vi "Three_Tote_was_working_ok.vi"(11 "3_Tote_Enable":bool=TRUE) -> ()   [LabVIEW 2014]
uses:
  General_VI/Global Var.vi
panel:
  in  "Time _To_Drive_1_Tote":i32=8000
  in  "Extend_Flipper_Time":i32=500
  in  "Open_Infeed_time":i32=800
  # "Static Tunning Values"
  # "extend flipper arm was 500"
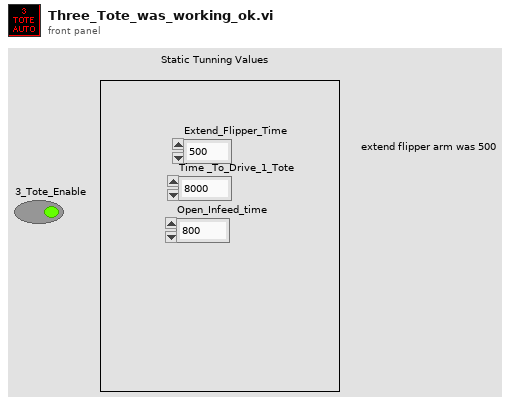
[diagram p1: front panel]
types:
  T1 = cluster{"Open_Infeed_time":i32, "Extend_Flipper_Time":i32, "Time _To_Drive_1_Tote":i32}
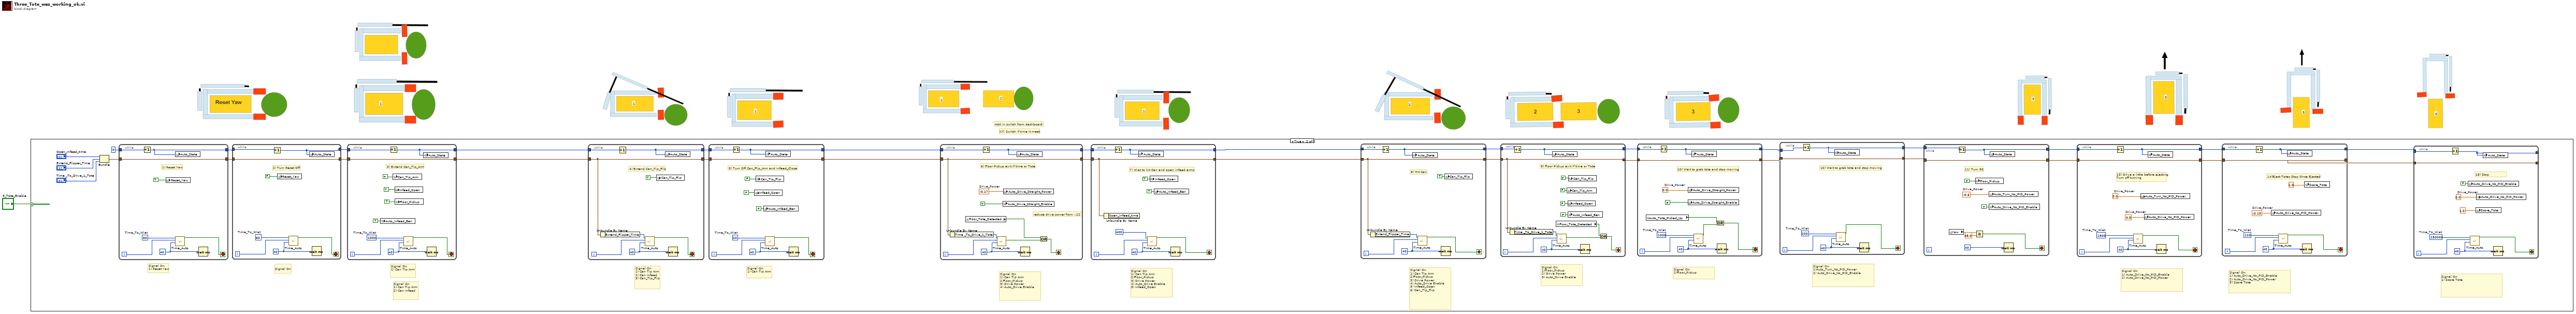
[diagram p0: block diagram]
diagram:
  # "3"
  # "3"
  # "3"
  # "3"
  # "2"
  # "2"
  # "2"
  # "1"
  # "1"
  # "1"
  # "1"
  # "Add in switch from dashboard"
  # "Kill Switch if time it meet"
  n1 = case shown="True" "3_Tote_Enable" {
    frame False {
    }
    frame True {
      # "Signal On\n1) Score Tote"
      # "Signal On\n1) Auto_Drive_No_PID_Enable\n2) Auto_Drive_No_PID_Power\n3) Score Tote"
      # "Signal On\n1) Auto_Drive_No_PID_Enable\n2) Auto_Drive_No_PID_Power"
      # "Signal On\n1)Auto_Turn_No_PID_Power\n2) Auto_Drive_No_PID_Enable"
      # "Signal On\n1)Floor_Pickup"
      # "Signal On\n1)Floor_Pickup\n2) Drive Power\n3) Auto_Drive Enable"
      # "Signal On\n1) Can Tip Arm\n2)Floor_Pickup\n3) Drive Power\n4) Auto_Drive Enable\n5) Infeed_Open\n6) Can_Tip_Flip"
      # "Signal On\n1) Can Tip Arm\n2)Floor_Pickup\n3) Drive Power\n4) Auto_Drive Enable\n5) Infeed_Open"
      # "Signal On\n1) Can Tip Arm\n2)Floor_Pickup\n3) Drive Power\n4) Auto_Drive Enable"
      # "Signal On\n1) Can Tip Arm"
      # "Signal On\n1) Can Tip Arm\n2) Can Infeed\n3) Can_Tip_Flip"
      # "Signal On\n1) Can Tip Arm\n2) Can Infeed"
      # "Signal On\n1) Can Tip Arm"
      # "Signal On"
      # "Signal On\n1) Reset Yaw"
      n2 = Bundle("Open_Infeed_time"="Open_Infeed_time", "Extend_Flipper_Time"="Extend_Flipper_Time", "Time _To_Drive_1_Tote"="Time _To_Drive_1_Tote") -> (w19:T1)  [unwired: 1 in]
      n3 = while {
        tunnel: 0 -> [w170]
        tunnel: [w169] -> w33
        tunnel: w19 -> [w171]
        tunnel: [w171] -> w18
        i -> [w174]
        stop <- w176 stop-if-true
        w175 = u32 40 ("milliseconds to wait")
        w173 = 60  # Time_To_Wiat
        # "1) Reset Yaw"
        n4 = Increment(x=w170) -> (x+1=w169:i32)
        n5 = global write "Global Var.vi" "Reset_Yaw"(TRUE) -> ()
        n6 = global write "Global Var.vi" "Auto_State"(w169) -> ()
        n7 = call "Time_Auto.vi"("Sample_Time"=w175, "Counter"=w174, "Time_to_wait"=w173) -> ("Boolean"=w176:bool)  [unwired: 8 in]
        n8 = Wait (ms)(milliseconds to wait=w175) -> ()  [unwired: 1 out]
      }
      n9 = while {
        tunnel: w33 -> [w162]
        tunnel: [w161] -> w32
        tunnel: w18 -> [w163]
        tunnel: [w163] -> w17
        i -> [w166]
        stop <- w168 stop-if-true
        w167 = u32 40 ("milliseconds to wait")
        w165 = 60  # Time_To_Wiat
        # "2) Turn Reset Off"
        n10 = Increment(x=w162) -> (x+1=w161:i32)
        n11 = global write "Global Var.vi" "Reset_Yaw"(FALSE) -> ()
        n12 = call "Time_Auto.vi"("Sample_Time"=w167, "Counter"=w166, "Time_to_wait"=w165) -> ("Boolean"=w168:bool)  [unwired: 8 in]
        n13 = global write "Global Var.vi" "Auto_State"(w161) -> ()
        n14 = Wait (ms)(milliseconds to wait=w167) -> ()  [unwired: 1 out]
      }
      n15 = while {
        tunnel: w32 -> [w154]
        tunnel: [w153] -> w7
        tunnel: w17 -> [w155]
        tunnel: [w155] -> w6
        i -> [w158]
        stop <- w160 stop-if-true
        w159 = u32 40 ("milliseconds to wait")
        w157 = 1000  # Time_To_Wiat
        # "3) Extend Can_Tip_Arm"
        n16 = global write "Global Var.vi" "Auto_Infeed_Ben"(TRUE ("Auto_Infeed_Ben")) -> ()
        n17 = Increment(x=w154) -> (x+1=w153:i32)
        n18 = global write "Global Var.vi" "Can_Tip_Arm"(TRUE) -> ()
        n19 = global write "Global Var.vi" "Infeed_Open"(TRUE) -> ()
        n20 = global write "Global Var.vi" "Floor_Pickup"(TRUE) -> ()
        n21 = call "Time_Auto.vi"("Sample_Time"=w159, "Counter"=w158, "Time_to_wait"=w157) -> ("Boolean"=w160:bool)  [unwired: 8 in]
        n22 = global write "Global Var.vi" "Auto_State"(w153) -> ()
        n23 = Wait (ms)(milliseconds to wait=w159) -> ()  [unwired: 1 out]
      }
      n24 = while {
        tunnel: w7 -> [w145]
        tunnel: [w144] -> w31
        tunnel: w6 -> [w143]
        tunnel: [w143] -> w16
        i -> [w147]
        stop <- w149 stop-if-true
        w148 = u32 40 ("milliseconds to wait")
        # "4) Extend Can_Tip_Flip"
        n25 = Unbundle By Name(w143) -> ("Extend_Flipper_Time"=w142:i32)
        n26 = Increment(x=w145) -> (x+1=w144:i32)
        n27 = call "Time_Auto.vi"("Sample_Time"=w148, "Counter"=w147, "Time_to_wait"=w142) -> ("Boolean"=w149:bool)  [unwired: 8 in]
        n28 = global write "Global Var.vi" "Can_Tip_Flip"(TRUE) -> ()
        n29 = global write "Global Var.vi" "Auto_State"(w144) -> ()
        n30 = Wait (ms)(milliseconds to wait=w148) -> ()  [unwired: 1 out]
      }
      n31 = while {
        tunnel: w31 -> [w134]
        tunnel: [w133] -> w27
        tunnel: w16 -> [w135]
        tunnel: [w135] -> w15
        i -> [w139]
        stop <- w141 stop-if-true
        w140 = u32 40 ("milliseconds to wait")
        w138 = 20  # Time_To_Wiat
        # "5) Turn Off Can_Flip_Arm and Infeed_Close"
        n32 = Increment(x=w134) -> (x+1=w133:i32)
        n33 = global write "Global Var.vi" "Infeed_Open"(FALSE) -> ()
        n34 = global write "Global Var.vi" "Can_Tip_Flip"(FALSE) -> ()
        n35 = global write "Global Var.vi" "Auto_Infeed_Ben"(FALSE ("Auto_Infeed_Ben")) -> ()
        n36 = call "Time_Auto.vi"("Sample_Time"=w140, "Counter"=w139, "Time_to_wait"=w138) -> ("Boolean"=w141:bool)  [unwired: 8 in]
        n37 = global write "Global Var.vi" "Auto_State"(w133) -> ()
        n38 = Wait (ms)(milliseconds to wait=w140) -> ()  [unwired: 1 out]
      }
      n39 = while {
        tunnel: w27 -> [w127]
        tunnel: [w126] -> w30
        tunnel: w15 -> [w125]
        tunnel: [w125] -> w14
        i -> [w130]
        stop <- w129 stop-if-true
        w123 = -0.17  # Drive_Power
        w131 = u32 40 ("milliseconds to wait")
        # "reduce drive power from -.22"
        # "6) Floor Pickup exit if time or Tote"
        n40 = Unbundle By Name(w125) -> ("Time _To_Drive_1_Tote"=w124:i32)
        n41 = global read "Global Var.vi" "Floor_Tote_Detected"() -> (w121:bool)
        n42 = Increment(x=w127) -> (x+1=w126:i32)
        n43 = call "Time_Auto.vi"("Sample_Time"=w131, "Counter"=w130, "Time_to_wait"=w124) -> ("Boolean"=w128:bool)  [unwired: 8 in]
        n44 = global write "Global Var.vi" "Auto_Drive_Straight_Enable"(TRUE) -> ()
        n45 = global write "Global Var.vi" "Auto_Drive_Straight_Power"(w123) -> ()
        n46 = global write "Global Var.vi" "Auto_State"(w126) -> ()
        n47 = Wait (ms)(milliseconds to wait=w131) -> ()  [unwired: 1 out]
        n48 = Or(x=w121, y=w128) -> (x .or. y?=w129:bool)
      }
      n49 = while {
        tunnel: w30 -> [w116]
        tunnel: [w115] -> w26
        tunnel: w14 -> [w114]
        tunnel: [w114] -> w13
        i -> [w119]
        stop <- w118 stop-if-true
        w120 = u32 40 ("milliseconds to wait")
        # "7) Wiat to hit Can and open infeed arms"
        n50 = Unbundle By Name(w114) -> ()  [unwired: 1 out]
        n51 = Increment(x=w116) -> (x+1=w115:i32)
        n52 = global write "Global Var.vi" "Auto_State"(w115) -> ()
        n53 = call "Time_Auto.vi"("Sample_Time"=w120, "Counter"=w119, "Time_to_wait"=u32 400 ("milliseconds to wait")) -> ("Boolean"=w118:bool)  [unwired: 8 in]
        n54 = global write "Global Var.vi" "Infeed_Open"(TRUE ("Infeed_Open")) -> ()
        n55 = global write "Global Var.vi" "Auto_Infeed_Ben"(TRUE ("Auto_Infeed_Ben")) -> ()
        n56 = Wait (ms)(milliseconds to wait=w120) -> ()  [unwired: 1 out]
      }
      n57 = while {
        tunnel: w26 -> [w107]
        tunnel: [w106] -> w29
        tunnel: w13 -> [w105]
        tunnel: [w105] -> w12
        i -> [w110]
        stop <- w109 stop-if-true
        w111 = u32 40 ("milliseconds to wait")
        # "8) HIt Can"
        n58 = Unbundle By Name(w105) -> ("Extend_Flipper_Time"=w104:i32)
        n59 = Increment(x=w107) -> (x+1=w106:i32)
        n60 = global write "Global Var.vi" "Auto_State"(w106) -> ()
        n61 = call "Time_Auto.vi"("Sample_Time"=w111, "Counter"=w110, "Time_to_wait"=w104) -> ("Boolean"=w109:bool)  [unwired: 8 in]
        n62 = Wait (ms)(milliseconds to wait=w111) -> ()  [unwired: 1 out]
        n63 = global write "Global Var.vi" "Can_Tip_Flip"(TRUE ("Infeed_Open")) -> ()
      }
      n64 = while {
        tunnel: w29 -> [w95]
        tunnel: [w94] -> w28
        tunnel: w12 -> [w92]
        tunnel: [w92] -> w11
        i -> [w102]
        stop <- w101 stop-if-true
        w103 = u32 40 ("milliseconds to wait")
        # "9) Floor Pickup exit if time or Tote"
        n65 = Unbundle By Name(w92) -> ("Time _To_Drive_1_Tote"=w93:i32)
        n66 = Increment(x=w95) -> (x+1=w94:i32)
        n67 = global write "Global Var.vi" "Auto_State"(w94) -> ()
        n68 = global read "Global Var.vi" "Floor_Tote_Detected"() -> (w99:bool)
        n69 = call "Time_Auto.vi"("Sample_Time"=w103, "Counter"=w102, "Time_to_wait"=w93) -> ("Boolean"=w100:bool)  [unwired: 8 in]
        n70 = global write "Global Var.vi" "Can_Tip_Arm"(FALSE ("Infeed_Open")) -> ()
        n71 = global write "Global Var.vi" "Infeed_Open"(FALSE ("Infeed_Open")) -> ()
        n72 = global write "Global Var.vi" "Auto_Infeed_Ben"(FALSE ("Auto_Infeed_Ben")) -> ()
        n73 = global write "Global Var.vi" "Can_Tip_Flip"(FALSE ("Infeed_Open")) -> ()
        n74 = Wait (ms)(milliseconds to wait=w103) -> ()  [unwired: 1 out]
        n75 = Or(x=w99, y=w100) -> (x .or. y?=w101:bool)
      }
      n76 = while {
        tunnel: w28 -> [w86]
        tunnel: [w85] -> w5
        tunnel: w11 -> [w87]
        tunnel: [w87] -> w3
        i -> [w89]
        stop <- w80 stop-if-true
        w84 = 0.0  # Drive_Power
        w90 = u32 40 ("milliseconds to wait")
        w88 = 1000  # Time_To_Wiat
        # "10) Wait to grab tote and stop moving"
        n77 = global read "Global Var.vi" "Auto_Tote_Picked_Up"() -> (w82:bool)
        n78 = Increment(x=w86) -> (x+1=w85:i32)
        n79 = global write "Global Var.vi" "Auto_Drive_Straight_Enable"(FALSE) -> ()
        n80 = global write "Global Var.vi" "Auto_Drive_Straight_Power"(w84) -> ()
        n81 = global write "Global Var.vi" "Auto_State"(w85) -> ()
        n82 = call "Time_Auto.vi"("Sample_Time"=w90, "Counter"=w89, "Time_to_wait"=w88) -> ("Boolean"=w81:bool)  [unwired: 8 in]
        n83 = Or(x=w82, y=w81) -> (x .or. y?=w80:bool)
        n84 = Wait (ms)(milliseconds to wait=w90) -> ()  [unwired: 1 out]
      }
      n85 = while {
        tunnel: w5 -> [w37]
        tunnel: [w36] -> w4
        tunnel: w3 -> [w38]
        tunnel: [w38] -> w2
        i -> [w40]
        stop <- w35 stop-if-true
        w41 = u32 40 ("milliseconds to wait")
        w39 = 200  # Time_To_Wiat
        # "10) Wait to grab tote and stop moving"
        n86 = Increment(x=w37) -> (x+1=w36:i32)
        n87 = global write "Global Var.vi" "Auto_State"(w36) -> ()
        n88 = call "Time_Auto.vi"("Sample_Time"=w41, "Counter"=w40, "Time_to_wait"=w39) -> ("Boolean"=w35:bool)  [unwired: 8 in]
        n89 = Wait (ms)(milliseconds to wait=w41) -> ()  [unwired: 1 out]
      }
      n90 = while {
        tunnel: [w73] -> w25
        tunnel: w2 -> [w74]
        tunnel: [w74] -> w10
        tunnel: w4 -> [w70]
        stop <- w75 stop-if-true
        w72 = -0.6  # Drive_Power
        # "11) Turn 90"
        n91 = global read "Global Var.vi" "Yaw"() -> (w77:dbl)
        n92 = Increment(x=w70) -> (x+1=w73:i32)
        n93 = Greater Or Equal?(x=w77, y=48.0) -> (x >= y?=w75:bool)
        n94 = global write "Global Var.vi" "Floor_Pickup"(FALSE) -> ()
        n95 = global write "Global Var.vi" "Auto_Turn_No_PID_Power"(w72) -> ()
        n96 = global write "Global Var.vi" "Auto_Drive_No_PID_Enable"(TRUE ("Auto_Drive_No_PID_Enable")) -> ()
        n97 = global write "Global Var.vi" "Auto_State"(w73) -> ()
        n98 = Wait (ms)(milliseconds to wait=u32 40) -> ()  [unwired: 1 out]
      }
      n99 = while {
        tunnel: w25 -> [w63]
        tunnel: [w62] -> w24
        tunnel: w10 -> [w64]
        tunnel: [w64] -> w9
        i -> [w68]
        stop <- w66 stop-if-true
        w61 = 0.0  # Drive_Power
        w65 = 0.5  # Drive_Power
        w69 = u32 40 ("milliseconds to wait")
        w67 = 1900  # Time_To_Wiat
        # "13) Drive a little before ejecting\nTurn off turning"
        n100 = Increment(x=w63) -> (x+1=w62:i32)
        n101 = call "Time_Auto.vi"("Sample_Time"=w69, "Counter"=w68, "Time_to_wait"=w67) -> ("Boolean"=w66:bool)  [unwired: 8 in]
        n102 = global write "Global Var.vi" "Auto_Turn_No_PID_Power"(w61) -> ()
        n103 = global write "Global Var.vi" "Auto_Drive_No_PID_Power"(w65) -> ()
        n104 = global write "Global Var.vi" "Auto_State"(w62) -> ()
        n105 = Wait (ms)(milliseconds to wait=w69) -> ()  [unwired: 1 out]
      }
      n106 = while {
        tunnel: w24 -> [w54]
        tunnel: [w53] -> w23
        tunnel: w9 -> [w55]
        tunnel: [w55] -> w8
        i -> [w59]
        stop <- w57 stop-if-true
        w52 = -0.15  # Drive_Power
        w60 = u32 40 ("milliseconds to wait")
        w58 = 120  # Time_To_Wiat
        # "14)Eject Totes Stop Once Ejected"
        n107 = Increment(x=w54) -> (x+1=w53:i32)
        n108 = global write "Global Var.vi" "Auto_Drive_No_PID_Power"(w52) -> ()
        n109 = call "Time_Auto.vi"("Sample_Time"=w60, "Counter"=w59, "Time_to_wait"=w58) -> ("Boolean"=w57:bool)  [unwired: 8 in]
        n110 = global write "Global Var.vi" "Auto_State"(w53) -> ()
        n111 = Wait (ms)(milliseconds to wait=w60) -> ()  [unwired: 1 out]
        n112 = global write "Global Var.vi" "Score_Tote"(1.0) -> ()
      }
      n113 = while {
        tunnel: w23 -> [w45]
        tunnel: w8 -> [w46]
        tunnel: [w46] -> _
        tunnel: [w44] -> _
        i -> [w50]
        stop <- w48 stop-if-true
        w42 = 0.0  # Drive_Power
        w51 = u32 40 ("milliseconds to wait")
        w49 = 150000  # Time_To_Wiat
        # "15) Stop"
        n114 = Increment(x=w45) -> (x+1=w44:i32)
        n115 = global write "Global Var.vi" "Auto_Drive_No_PID_Enable"(FALSE ("Auto_Drive_No_PID_Enable")) -> ()
        n116 = call "Time_Auto.vi"("Sample_Time"=w51, "Counter"=w50, "Time_to_wait"=w49) -> ("Boolean"=w48:bool)  [unwired: 8 in]
        n117 = global write "Global Var.vi" "Score_Tote"(1.0) -> ()
        n118 = global write "Global Var.vi" "Auto_Drive_No_PID_Power"(w42) -> ()
        n119 = global write "Global Var.vi" "Auto_State"(w44) -> ()
        n120 = Wait (ms)(milliseconds to wait=w51) -> ()  [unwired: 1 out]
      }
    }
  }
